vi "Set ScriptDatabase.vi"(8 "error in (no error)":errorcluster, 10 "ScriptDatabase":refnum<class "ScriptDatabase.lvclass">, 11 "ScriptsConfiguration in":refnum<class "ScriptSetting.lvclass">) -> (0 "error out":errorcluster, 3 "ScriptsConfiguration out":refnum<class "ScriptSetting.lvclass">)   [LabVIEW 2015, in "ScriptSetting.lvclass"]
uses:
  ScriptSetting.lvclass
  _Database/Implements/ScriptDatabase.lvclass
  ScriptSetting.lvclass/ScriptSetting.ctl
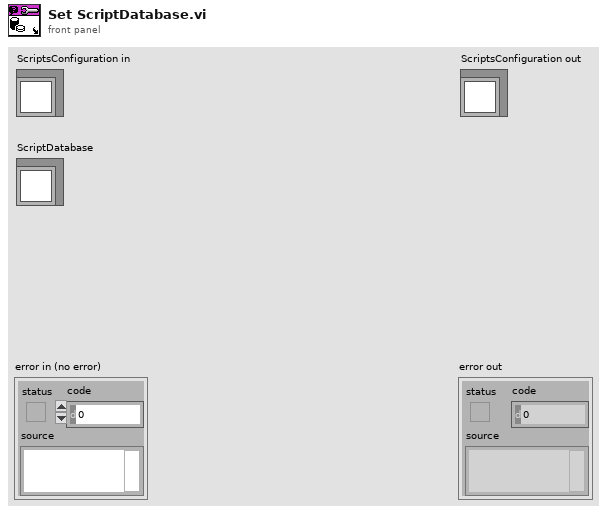
[diagram p1: front panel]
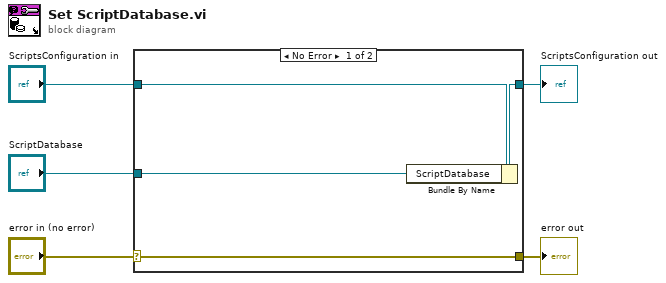
[diagram p0: block diagram]
diagram:
  n1 = case shown="No Error" "error in (no error)" {
    selector: "error in (no error)" -> [w9 w10]
    tunnel: [w9 w10] -> w4
    tunnel: [w7 w11] -> w2
    tunnel: "ScriptsConfiguration in" -> [w8 w11]
    tunnel: "ScriptDatabase" -> [w6 _]
    frame No Error {
      n2 = Bundle By Name(cluster=w8, "ScriptDatabase"=w6) -> (w7:refnum<class "ScriptSetting.lvclass">)
    }
    frame Error {
    }
  }
  "error out" <- w4
  "ScriptsConfiguration out" <- w2
